vi "Read Command Words.vi"(8 "error in":errorcluster, 11 "Execution Unit in":refnum<class "Execution Unit.lvclass">) -> (0 "error out":errorcluster, 2 "command words":T1[](array[typedef]), 3 "Execution Unit out":refnum<class "Execution Unit.lvclass">)   [LabVIEW 2020, in "Ballard MIL-STD-1553 Engine.lvlib" / "Implementation.lvlib" / "Execution Unit.lvclass"]
uses:
  Execution Unit.lvclass
  Shared/Command Word.ctl
  Execution Unit.lvclass/Execution Unit.ctl
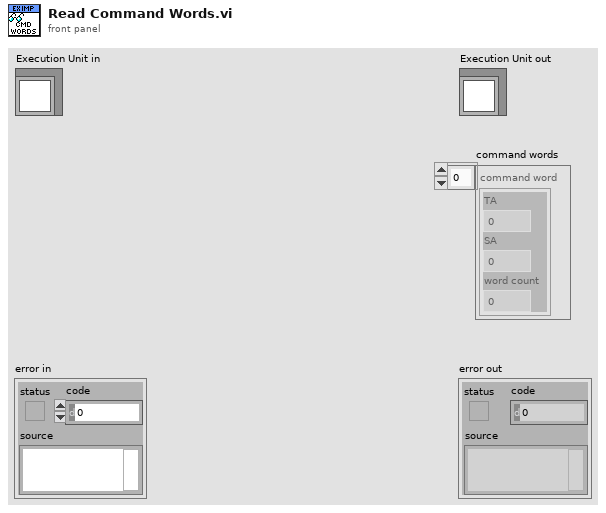
[diagram p1: front panel]
types:
  T1 = typedef "Command Word.ctl" = cluster{"TA":i8, "SA":i8, "word count":i8}
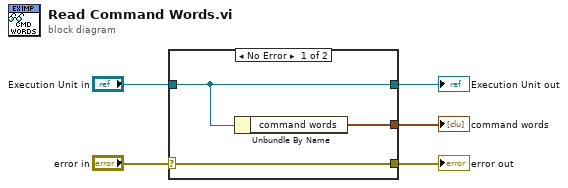
[diagram p0: block diagram]
diagram:
  n1 = case shown="No Error" "error in" {
    selector: "error in" -> [w8 w9]
    tunnel: [w8 w9] -> w4
    tunnel: [w7 w10] -> w2
    tunnel: "Execution Unit in" -> [w7 w10]
    tunnel: [w6 _] -> w1
    frame No Error {
      n2 = Unbundle By Name(w7) -> ("command words"=w6:T1[])
    }
    frame Error {
    }
  }
  "error out" <- w4
  "Execution Unit out" <- w2
  "command words" <- w1
